vi "Routine to Side.vi"(11 "Routines":T1) -> (2 "Scale Side":T2, 3 "Switch Side":T2)   [LabVIEW 2017]
uses:
  Side.ctl
  Routines.ctl
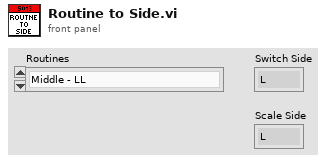
[diagram p1: front panel]
types:
  T1 = typedef "Routines.ctl" = enum16{"Middle - LL", "Middle - LR", "Middle - RL", "Middle - RR", "Far Right - LL", "Far Right - LR", "Far Right - RL", "Far Right - RR", "Far Left - LL", "Far Left - LR", "Far Left - RL", "Far Left - RR"}
  T2 = typedef "Side.ctl" = enum16{"L", "R"}
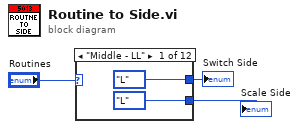
[diagram p0: block diagram]
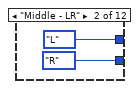
[diagram p2: hidden frame]
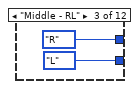
[diagram p3: hidden frame]
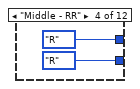
[diagram p4: hidden frame]
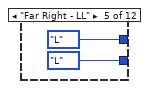
[diagram p5: hidden frame]
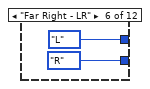
[diagram p6: hidden frame]
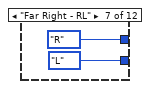
[diagram p7: hidden frame]
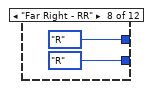
[diagram p8: hidden frame]
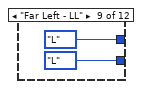
[diagram p9: hidden frame]
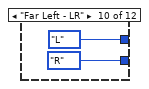
[diagram p10: hidden frame]
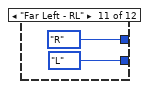
[diagram p11: hidden frame]
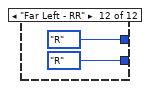
[diagram p12: hidden frame]
diagram:
  n1 = case shown="\"Middle - LL\"" "Routines" {
    tunnel: [Side."L" ("Side") Side."L" ("Side") Side."R" ("Side") Side."R" ("Side") Side."L" ("Side") Side."L" ("Side") Side."R" ("Side") Side."R" ("Side") Side."L" ("Side") Side."L" ("Side") Side."R" ("Side") Side."R" ("Side")] -> w2
    tunnel: [Side."L" ("Side") Side."R" ("Side") Side."L" ("Side") Side."R" ("Side") Side."L" ("Side") Side."R" ("Side") Side."L" ("Side") Side."R" ("Side") Side."L" ("Side") Side."R" ("Side") Side."L" ("Side") Side."R" ("Side")] -> w3
    frame "Middle - LL" {
    }
    frame "Middle - LR" {
    }
    frame "Middle - RL" {
    }
    frame "Middle - RR" {
    }
    frame "Far Right - LL" {
    }
    frame "Far Right - LR" {
    }
    frame "Far Right - RL" {
    }
    frame "Far Right - RR" {
    }
    frame "Far Left - LL" {
    }
    frame "Far Left - LR" {
    }
    frame "Far Left - RL" {
    }
    frame "Far Left - RR" {
    }
  }
  "Scale Side" <- w3
  "Switch Side" <- w2
